vi "poly_process_api_vi_ref_pre.vi"(7 "name of caller in (you)":string, 8 "error in":errorcluster, 9 "vi path":path, 10 "api vi ref in":T1) -> (0 "error out":errorcluster, 2 "api vi ref out":T1)   [LabVIEW 2015]
uses:
  api_vi_ref.ctl
  error_tools/error_handler.vi
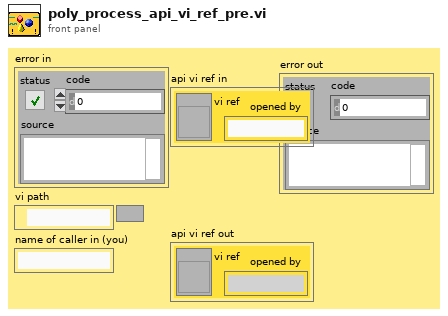
[diagram p1: front panel]
types:
  T1 = typedef "api_vi_ref.ctl" = cluster{"vi ref":refnum<vi>, "opened by":string}
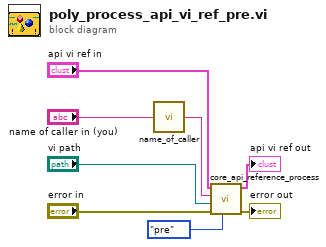
[diagram p0: block diagram]
diagram:
  n1 = call "name_of_caller.vi"("name of caller in"="name of caller in (you)") -> ("name of caller out"=w2:string)  [unwired: 3 in]
  n2 = call "core_api_reference_process.vi"("pre/post"=enum16{"pre", "post"}."pre" ("pre/post (pre)"), "error in"="error in", "vi path"="vi path", "name of caller in"=w2, "api vi ref in"="api vi ref in") -> ("error out"=→"error out":errorcluster, "api vi ref out"=→"api vi ref out":T1)  [unwired: 5 in]
